vi "connect to pulsator.vi"(8 "comms in":T2, 10 "message scheduler":refnum<class "message scheduler.lvclass">, 11 "queues":T1) -> (0 "comms out":T2)   [LabVIEW 2018]
uses:
  type defs/comms loop data.ctl
  ICL-LabVIEW_General/Incident logger/Incident logger.lvclass
  <vilib>/Modbus/master/Modbus Master.lvclass
  type defs/Queues.ctl
  ICL-LabVIEW_General/Message Scheduler/message scheduler.lvclass
  ICL-LabVIEW_General/Message Scheduler/generic message queue/standard message queue/standard message.lvclass
  C:/GitHub/ICL-LabVIEW_General/Message Scheduler/generic message queue/generic message.lvclass
  <vilib>/Modbus/master/Create Master Instance (TCP).vi
  ICL-LabVIEW_General/Pulser Controller/AKD MODBUS commands/enable drive.vi
  ICL-LabVIEW_General/Pulser Controller/AKD MODBUS commands/home.vi
  <vilib>/Utility/error.llb/Error Cluster From Error Code.vi
  <vilib>/ErrorRing/Error Ring.xnode
  ICL-LabVIEW_General/Pulser Controller/Pulser controller commands library.lvlib
  ICL-LabVIEW_General/Message Scheduler/scheduled message/scheduled message.lvclass
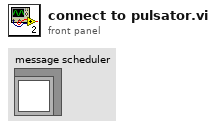
[diagram p1: front panel]
types:
  T1 = typedef "Queues.ctl" = cluster{"messageHandler":refnum<queue>, "comms":refnum<queue>, "dataStream":refnum<queue>, "dataProcessor":refnum<queue>, "fileIO":refnum<queue>, "userInterface":refnum<queue>, "errors":refnum<queue>, "customCompressor":refnum<queue>}
  T2 = typedef "comms loop data.ctl" = cluster{"params":cluster{"commandStream":cluster{"reader name":string, "writer name":string, "stream buffer size":i32}, "errorStream":cluster{"reader name":string, "writer name":string, "stream buffer size":i32}, "RT IP address":string, "pulserControllerIP":string}, "vars":cluster{"commandStream":refnum<k21>, "Incident logger":refnum<class "Incident logger.lvclass">, "check error scheduled message":u32, "errorStream":refnum<k21>, "watchdogScheduleID":u32, "pulsator":cluster{"pulser connection":refnum<class "Modbus Master.lvclass">, "pulserConnected":bool, "pulsatorScheduleID":u32, "pulserRunning":bool}}}
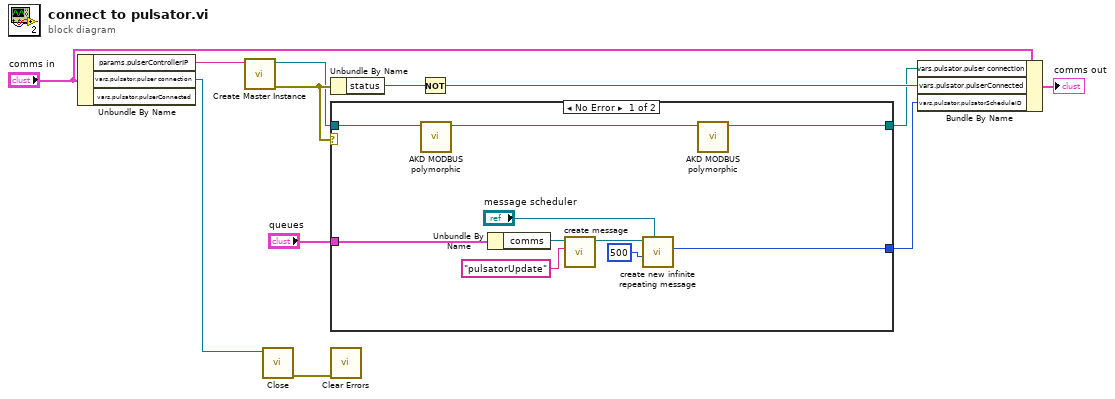
[diagram p0: block diagram]
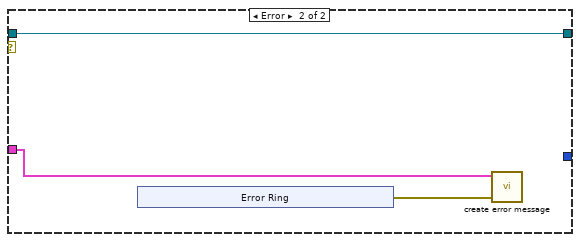
[diagram p2: hidden frame]
diagram:
  n1 = Unbundle By Name("comms in") -> ("params.pulserControllerIP"=w1:string, "vars.pulsator.pulser connection"=w10:refnum<class "Modbus Master.lvclass">)  [unwired: 1 out]
  n2 = call-poly <vilib>:"Create Master Instance.vi"("address"=w1) -> ("error out"=w6:errorcluster, "TCP master instance"=w5:refnum<class "Modbus Master.lvclass">)  [unwired: 9 in]
  n3 = call-dynamic "Close.vi"("Modbus master in"=w10) -> ("error out"=w9:errorcluster)  [unwired: 10 in]
  n4 = Unbundle By Name(w6) -> ("status"=w7:bool)
  n5 = case shown="No Error" w6 {
    tunnel: w5 -> [w22 w24]
    tunnel: [w20 w24] -> w4
    tunnel: "queues" -> [w19 w23]
    tunnel: [w13 _] -> w2
    frame No Error {
      n6 = call-poly "AKD MODBUS polymorphic.vi"("Modbus Master in"=w22) -> ("Modbus Master out"=w21:refnum<class "Modbus Master.lvclass">)  [unwired: 9 in, 1 out]
      n7 = Unbundle By Name(w19) -> ("comms"=w18:refnum<queue>)
      n8 = call "create message.vi"("message"="pulsatorUpdate", "queue ref"=w18) -> ("standard message out"=w16:refnum<class "standard message.lvclass">)  [unwired: 8 in, 1 out]
      n9 = call "create new infinite repeating message.vi"("message scheduler"="message scheduler", "ms delay"=u32 500, "message"=w16) -> ("schedule ID"=w13:u32)  [unwired: 7 in, 1 out]
      n10 = call-poly "AKD MODBUS polymorphic.vi"("Modbus Master in"=w21) -> ("Modbus Master out"=w20:refnum<class "Modbus Master.lvclass">)  [unwired: 10 in]
    }
    frame Error {
      n11 = xnode "Error Ring"() -> ("error out"=w25:errorcluster)
      n12 = call "create error message.vi"("error in (no error)"=w25, "queues"=w23) -> ()  [unwired: 10 in]
    }
  }
  n13 = call <vilib>:"Clear Errors.vi"("error in (no error)"=w9) -> ()  [unwired: 5 in, 2 out]
  n14 = Not(x=w7) -> (.not. x?=w8:bool)
  n15 = Bundle By Name(cluster="comms in", "vars.pulsator.pulser connection"=w4, "vars.pulsator.pulserConnected"=w8, "vars.pulsator.pulsatorScheduleID"=w2) -> (→"comms out":T2)
